vi "Publisher Do.vi"(8 "error in (no error)":errorcluster, 10 "Publisher in":refnum<class "Publisher.lvclass">, 11 "Subscribe Msg":refnum<class "Subscribe Msg.lvclass">) -> (0 "error out":errorcluster, 2 "Publisher out":refnum<class "Publisher.lvclass">)   [LabVIEW 2020, in "Publisher.lvlib" / "Subscribe Msg.lvclass"]
doc: "This VI delivers the message to the actor by calling the appropriate method(s) on the actor."
uses:
  Subscribe Msg.lvclass
  C:/Current projects/WS/Framework/Framework/Actors/Publisher/Publisher Messages/Publisher Msg/Publisher Msg.lvclass
  Publisher/Publisher.lvclass
  Publisher Msg/Publisher Msg.lvclass/Publisher Msg.ctl
  Subscribe Msg.lvclass/Subscribe Msg.ctl
  Publisher Msg/Publisher Msg.lvclass
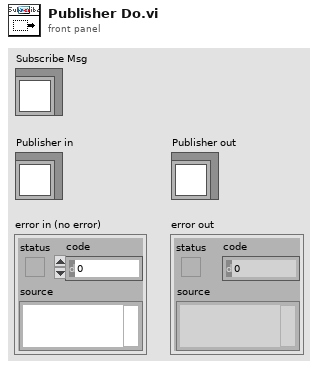
[diagram p1: front panel]
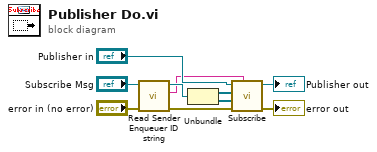
[diagram p0: block diagram]
diagram:
  n1 = call "Read Sender Enqueuer ID string.vi"("error in (no error)"="error in (no error)", "Publisher Msg in"="Subscribe Msg") -> ("error out"=w2:errorcluster, "Sender Enqueuer ID string"=w3:string, "Publisher Msg out"=w4:refnum<class "Subscribe Msg.lvclass">)  [unwired: 7 in]
  n2 = Unbundle(w4) -> (w8:refnum<class "Message.lvclass">[], w7:refnum<class "Data.lvclass">[])
  n3 = call "Subscribe.vi"("Enqueuer ID string"=w3, "error in (no error)"=w2, "Data Array"=w7, "Message Array"=w8, "Publisher in"="Publisher in") -> ("error out"=→"error out":errorcluster, "Publisher out"=→"Publisher out":refnum<class "Publisher.lvclass">)  [unwired: 4 in, 1 out]
